vi "WPI_PWMSetPeriodMultiplier.vi"(8 "error in (no error)":errorcluster, 10 "PWMPeriodMultiplier":T1 items=["1X"=0, "2X"=1, "4X"=3], 11 "PWMDeviceRef":T2={"DeviceStatus"={"status"=FALSE, "code"=0, "source"=""}, "PWM Channel"=enum."PWM 4"}) -> (0 "error out":errorcluster, 3 "PWMDeviceRef":T2={"DeviceStatus"={"status"=FALSE, "code"=0, "source"=""}, "PWM Channel"=enum."PWM 4"})   [LabVIEW 2017]
doc: "Scales the period of the PWM you specify.\n\nThis software is licensed. Open the labview\\readme\\WPI Robotics Library Open Source License.txt file for more information."
uses:
  <vilib>/Rock Robotics/WPI/PWM/WPI_PWMDeviceRef.ctl
  <vilib>/Rock Robotics/SystemInterfaces/DIO/FPGA_DIOPWMChannel.ctl
  <vilib>/Rock Robotics/WPI/PWM/WPI_PWMPeriodMultiplier.ctl
  <vilib>/Rock Robotics/WPI/PWM/WPI_PWMChannelCacheOp.ctl
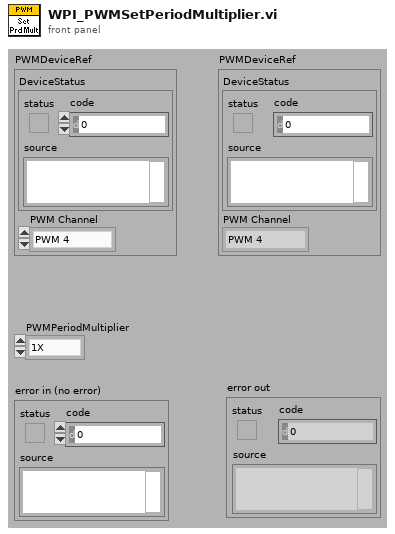
[diagram p1: front panel]
types:
  T1 = typedef "WPI_PWMPeriodMultiplier.ctl" = u8
  T2 = typedef "WPI_PWMDeviceRef.ctl" = cluster{"DeviceStatus":errorcluster, "PWM Channel":T3}
  T3 = typedef "FPGA_DIOPWMChannel.ctl" = enum8{"PWM 0", "PWM 1", "PWM 2", "PWM 3", "PWM 4", "PWM 5", "PWM 6", "PWM 7", "PWM 8", "PWM 9", "PWM MXP 0", "PWM MXP 1", "PWM MXP 2", "PWM MXP 3", "PWM MXP 4", "PWM MXP 5", "PWM MXP 6", "PWM MXP 7", "PWM MXP 8", "PWM MXP 9", "Invalid"}
  T4 = typedef "WPI_PWMChannelCacheOp.ctl" = enum16{"Acquire", "Release", "Status"}
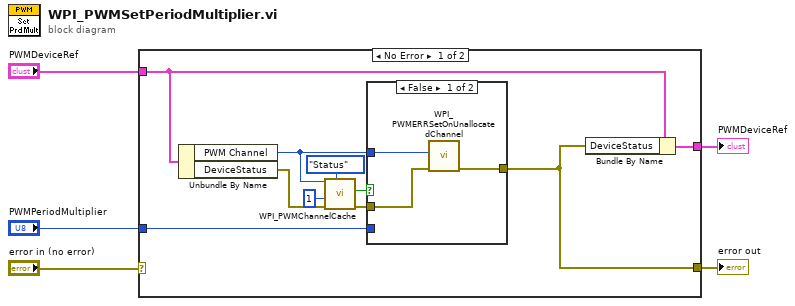
[diagram p0: block diagram]
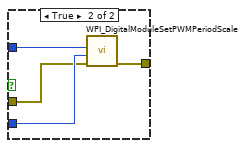
[diagram p2: hidden frame]
diagram:
  n1 = case shown="No Error" "error in (no error)" {
    selector: "error in (no error)" -> [_ w24]
    tunnel: "PWMDeviceRef" -> [w10 w23]
    tunnel: [w15 w23] -> w4
    tunnel: "PWMPeriodMultiplier" -> [w8 _]
    tunnel: [w7 w24] -> w2
    frame No Error {
      n2 = Unbundle By Name(w10) -> ("PWM Channel"=w9:T3, "DeviceStatus"=w14:errorcluster)
      n3 = call <vilib>:"WPI_PWMChannelCache.vi"("Operation"=WPI_PWMChannelCacheOp."Status", "error in (no error)"=w14, "Additional Depth"=1, "PWMChannel"=w9) -> ("error out"=w11:errorcluster, "Allocated?"=w12:bool)  [unwired: 1 in, 5 out]
      n4 = case shown="False" w12 {
        tunnel: [w17 w22] -> w7
        tunnel: w11 -> [w18 w19]
        tunnel: w9 -> [w16 w21]
        tunnel: w8 -> [_ w20]
        frame False {
          n5 = call <vilib>:"WPI_PWMERRSetOnUnallocatedChannel.vi"("error in (no error)"=w18, "PWM Channel"=w16) -> ("error out"=w17:errorcluster)  [unwired: 9 in]
        }
        frame True {
          n6 = call <vilib>:"WPI_DigitalModuleSetPWMPeriodScale.vi"("error in (no error)"=w19, "PeriodScale"=w20, "PWMChannel"=w21) -> ("error out"=w22:errorcluster)  [unwired: 2 in, 6 out]
        }
      }
      n7 = Bundle By Name(cluster=w10, "DeviceStatus"=w7) -> (w15:T2)
    }
    frame Error {
    }
  }
  "PWMDeviceRef" <- w4
  "error out" <- w2
